vi "CRYRecursive Tree.vi"(9 "pattern":string="*.vi", 10 "Sequence path":path, 11 "Tree in":refnum<vi>) -> (3 "Tree Out":refnum<vi>)   [LabVIEW 2013]
doc: "This VI uses a Tree Control to display the hierarchy of files and folders in a given directory. The VI searches first for subfolders of the directory, then for files with names that match a pattern you specify, such as *.vi. The VI displays the files and folders of the directory in hierarchical order in a Tree Control. \n\nNote: If you do not specify a pattern, the Tree Control displays all files except shortcuts."
panel:
  in  "Sequences":string(tree)
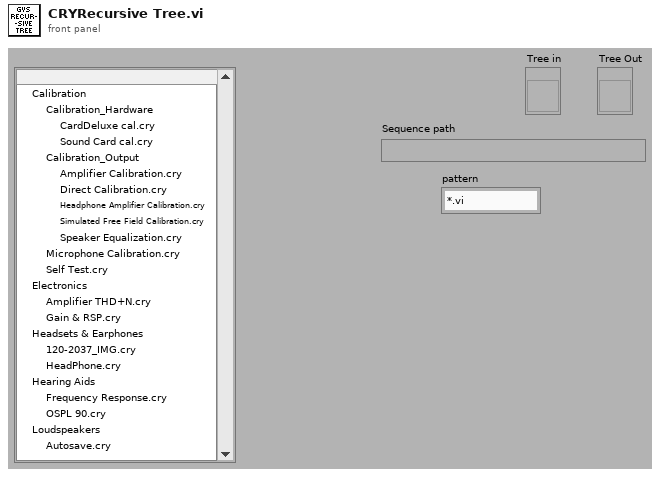
[diagram p1: front panel]
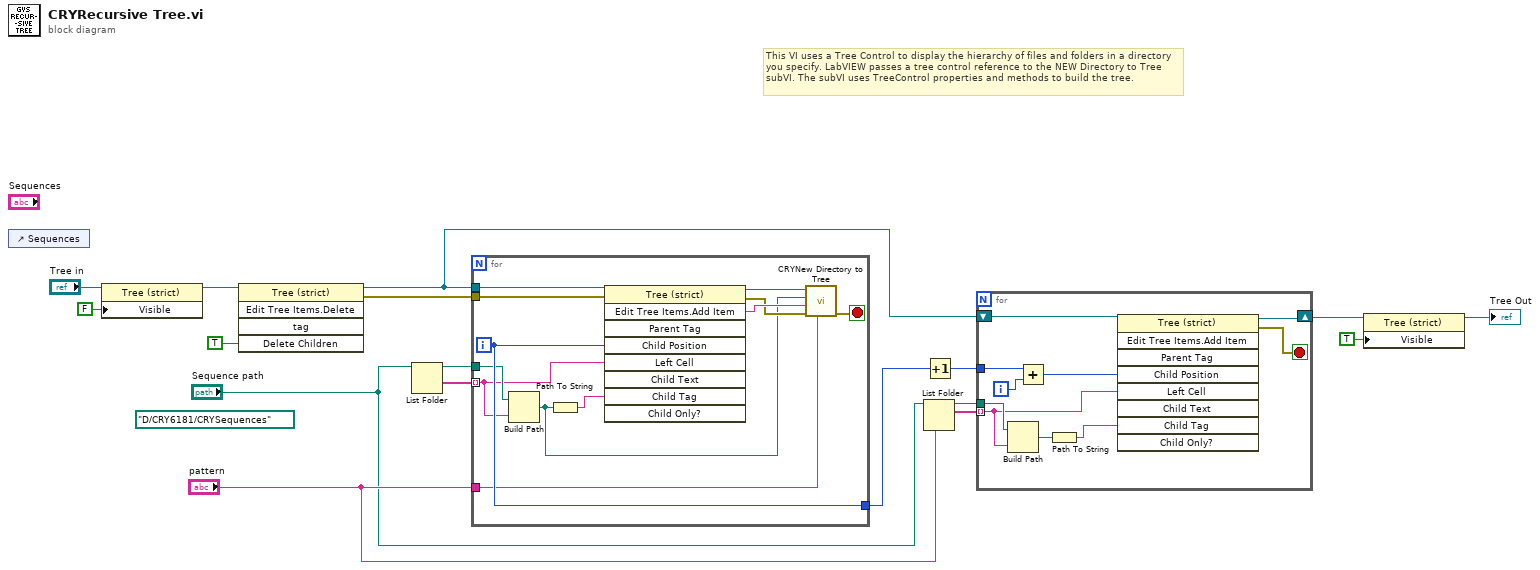
[diagram p0: block diagram]
diagram:
  (unwired) path "D:/CRY6181/CRYSequences" ("path")
  # "This VI uses a Tree Control to display the hierarchy of files and folders in a directory you specify. LabVIEW passes a tree control reference to the NEW Directory to Tree subVI. The subVI uses TreeControl properties and methods to build the tree."
  n1 = control-ref of="Sequences"() -> ()  [unwired: 1 out]
  n2 = property class="Tree (strict)"(reference="Tree in", "Visible"=FALSE) -> (reference out=w7:refnum<vi>)  [unwired: 1 in, 1 out]
  n3 = invoke class="Tree (strict)" method="Edit Tree Items.Delete"(reference=w7, "Delete Children"=TRUE ("Delete Children?")) -> (reference out=w12:refnum<vi>, error out=w16:errorcluster)  [unwired: 3 in, 3 out]
  n4 = List Folder(path="Sequence path") -> (path out=w9:path, folder names=w15:string[])  [unwired: 3 in, 2 out]
  n5 = for {
    tunnel: w12 -> [w29]
    tunnel: w16 -> [w28]
    tunnel: w15 -> [w20] mode=indexing
    tunnel: [w24] -> w13
    tunnel: "pattern" -> [w22]
    tunnel: w9 -> [w21]
    i -> [w24]
    stop <- w23 stop-if-true
    n6 = Build Path(base path=w21, name or relative path=w20) -> (appended path=w18:path)
    n7 = Path To String(path=w18) -> (string=w19:string)
    n8 = invoke class="Tree (strict)" method="Edit Tree Items.Add Item"(reference=w29, error in=w28, "Child Position"=w24, "Left Cell"=w20, "Child Tag"=w19) -> (reference out=w27:refnum<vi>, error out=w25:errorcluster, "Edit Tree Items:Add Item"=w26:string)  [unwired: 4 in, 6 out]
    n9 = call "CRYNew Directory to Tree.vi"("pattern"=w22, "error in"=w25, "Parent Tag"=w26, "directory path"=w18, "Tree"=w27) -> ("error out"=w23:errorcluster)  [unwired: 5 in, 1 out]
  }
  n10 = List Folder(path="Sequence path", pattern="pattern") -> (path out=w10:path, filenames=w14:string[])  [unwired: 2 in, 2 out]
  n11 = Increment(x=w13) -> (x+1=w3:i32)
  n12 = for {
    tunnel: w14 -> [w31] mode=indexing
    tunnel: w3 -> [w38]
    tunnel: w10 -> [w32]
    shift-right: [w34] -> w5
    shift-left: w12 -> [w39]
    i -> [w37]
    stop <- w35 stop-if-true
    n13 = Build Path(base path=w32, name or relative path=w31) -> (appended path=w33:path)
    n14 = Add(x=w38, y=w37) -> (x+y=w36:i32)
    n15 = Path To String(path=w33) -> (string=w30:string)
    n16 = invoke class="Tree (strict)" method="Edit Tree Items.Add Item"(reference=w39, "Child Position"=w36, "Left Cell"=w31, "Child Tag"=w30) -> (reference out=w34:refnum<vi>, error out=w35:errorcluster)  [unwired: 5 in, 7 out]
  }
  n17 = property class="Tree (strict)"(reference=w5, "Visible"=TRUE) -> (reference out=→"Tree Out":refnum<vi>)  [unwired: 1 in, 1 out]
